vi "Pointer.Read (I64).vi"(8 "error in (no error)":errorcluster, 11 "pointer in":u64) -> (0 "error out":errorcluster, 2 "value":i64, 3 "pointer out":u64)   [LabVIEW 2016, in "VeriStand Data.lvlib"]
doc: "Read a value from the provided <B>pointer</B>."
uses:
  VeriStand Data.lvlib
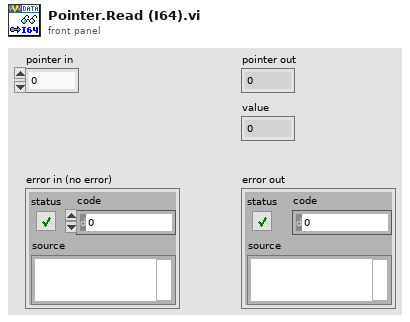
[diagram p1: front panel]
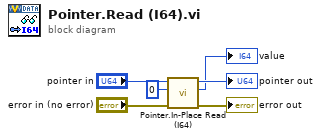
[diagram p0: block diagram]
diagram:
  n1 = call "Pointer.In-Place Read (I64).vi"("error in (no error)"="error in (no error)", "value in"=i64 0, "pointer in"="pointer in") -> ("error out"=→"error out":errorcluster, "value out"=→"value":i64, "pointer out"=→"pointer out":u64)  [unwired: 6 in]
